vi "Write TCP.vi"(8 "error in (no error)":errorcluster, 10 "TCP":refnum<class "TCP.lvclass">, 11 "MB_TCP in":refnum<class "MB_TCP.lvclass">) -> (0 "error out":errorcluster, 3 "MB_TCP out":refnum<class "MB_TCP.lvclass">)   [LabVIEW 2019, in "MB_TCP.lvclass"]
uses:
  MB_TCP.lvclass
  NI_modbus_upd/TCP/TCP.lvclass
  MB_TCP.lvclass/MB_TCP.ctl
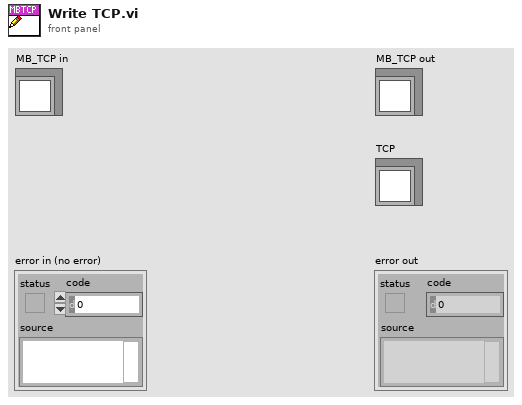
[diagram p1: front panel]
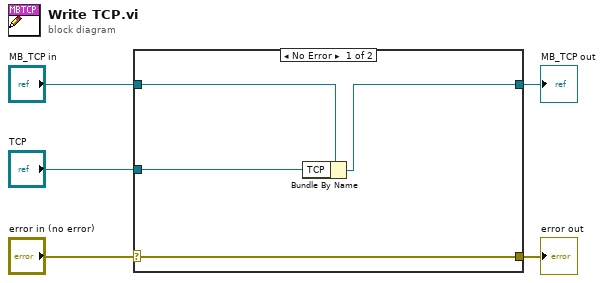
[diagram p0: block diagram]
diagram:
  n1 = case shown="No Error" "error in (no error)" {
    selector: "error in (no error)" -> [w9 w10]
    tunnel: [w9 w10] -> w4
    tunnel: [w6 w11] -> w2
    tunnel: "MB_TCP in" -> [w8 w11]
    tunnel: "TCP" -> [w7 _]
    frame No Error {
      n2 = Bundle By Name(cluster=w8, "TCP"=w7) -> (w6:refnum<class "MB_TCP.lvclass">)
    }
    frame Error {
    }
  }
  "error out" <- w4
  "MB_TCP out" <- w2
